vi "Sensors.vi"() -> ()   [LabVIEW 2018]
panel:
  out "Oil Pump":string
  out "Oil Pressure":string
  out "Chamber Temp":string
  out "Oil Temp":string
  out "Target Temp":string
  out "Vacuum":string
  out "-":string
  out "Recoat Temp":string
  out "Sprinkler Temp":string
  out "Overhead Temp":string
  out "Radiation Limit":string
  out "Recon Vars 2":string
  out "-":string
  out "Interlocks":string
  out "Solenoid A":string
  out "Solenoid B":string
  out "BOP 100-2ML":string
  out "Agilent 33120A":string
  out "- Grid Bias":string
  out "+ Grid Bias":string
  out "Cathode B":string
  out "Cathode C":string
  out "Cathode A":string
  out "Recon Vars":string
  out "Pulser C":string
  out "Pulser B":string
  out "Due MCU":string
  out "Pulser A":string
  out "Quantum 9530":string
  out "Beam Extraction":string
  out "Error":string
  out "Scanning Vars":string
  out "rPi Swivel Cam":string
  out "Port & Oil Cams":string
  out "Room Cams":string
  out "BeamAcceleration":string
  out "Sensors":string
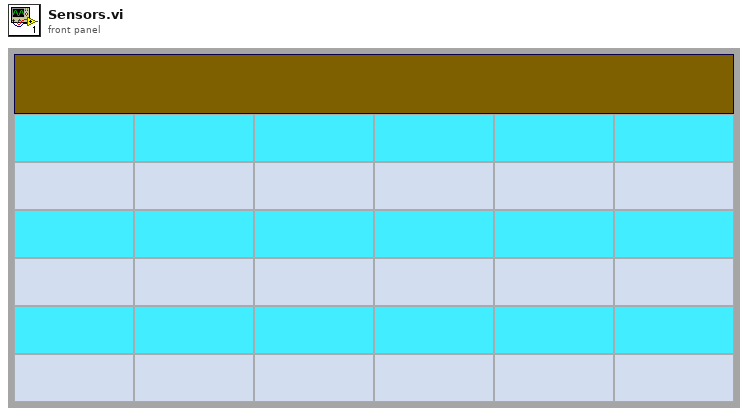
[diagram p1: front panel]
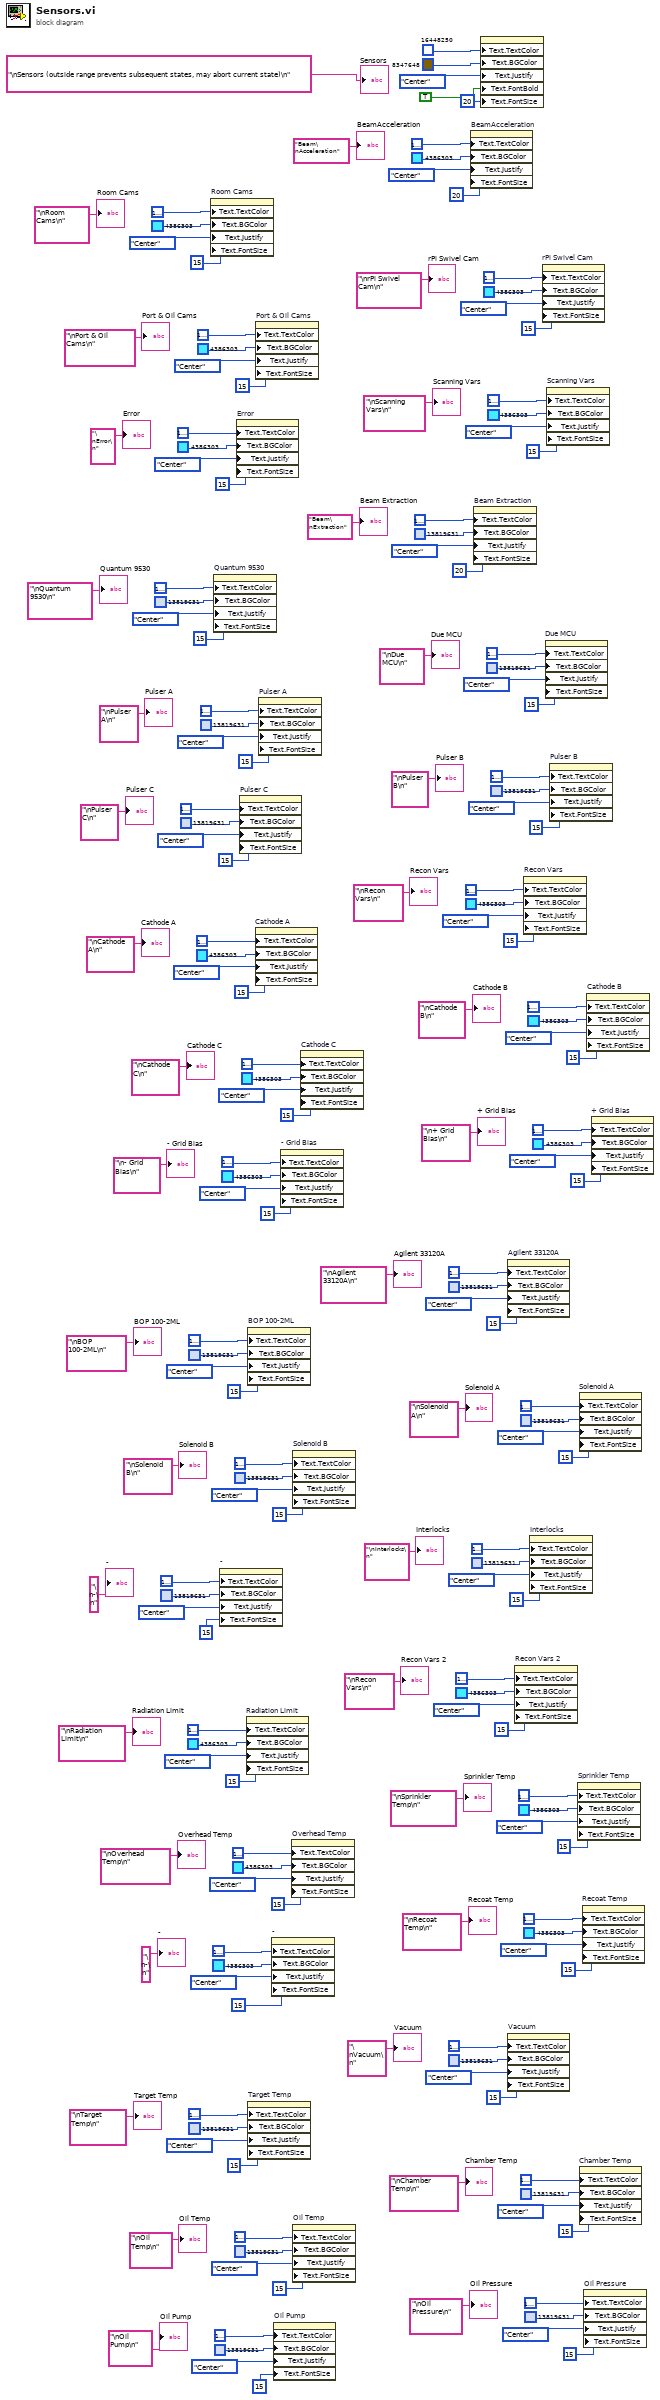
[diagram p0: block diagram]
diagram:
  n1 = property on="Room Cams" class="Str"("Text.TextColor"=u32 16777228, "Text.BGColor"=u32 4386303, "Text.Justify"=enum16{"Left", "Center", "Right"}."Center" ("Text.Justification"), "Text.FontSize"=u32 15 ("Text.Font:Size")) -> ()  [unwired: 2 in, 2 out]
  n2 = property on="Quantum 9530" class="Str"("Text.TextColor"=u32 16777228, "Text.BGColor"=u32 13819631, "Text.Justify"=enum16{"Left", "Center", "Right"}."Center" ("Text.Justification"), "Text.FontSize"=u32 15 ("Text.Font:Size")) -> ()  [unwired: 2 in, 2 out]
  n3 = property on="-" class="Str"("Text.TextColor"=u32 16777228, "Text.BGColor"=u32 13819631, "Text.Justify"=enum16{"Left", "Center", "Right"}."Center" ("Text.Justification"), "Text.FontSize"=u32 15 ("Text.Font:Size")) -> ()  [unwired: 2 in, 2 out]
  n4 = property on="Error" class="Str"("Text.TextColor"=u32 16777228, "Text.BGColor"=u32 4386303, "Text.Justify"=enum16{"Left", "Center", "Right"}."Center" ("Text.Justification"), "Text.FontSize"=u32 15 ("Text.Font:Size")) -> ()  [unwired: 2 in, 2 out]
  n5 = property on="Pulser C" class="Str"("Text.TextColor"=u32 16777228, "Text.BGColor"=u32 13819631, "Text.Justify"=enum16{"Left", "Center", "Right"}."Center" ("Text.Justification"), "Text.FontSize"=u32 15 ("Text.Font:Size")) -> ()  [unwired: 2 in, 2 out]
  n6 = property on="Radiation Limit" class="Str"("Text.TextColor"=u32 16777228, "Text.BGColor"=u32 4386303, "Text.Justify"=enum16{"Left", "Center", "Right"}."Center" ("Text.Justification"), "Text.FontSize"=u32 15 ("Text.Font:Size")) -> ()  [unwired: 2 in, 2 out]
  n7 = property on="BOP 100-2ML" class="Str"("Text.TextColor"=u32 16777228, "Text.BGColor"=u32 13819631, "Text.Justify"=enum16{"Left", "Center", "Right"}."Center" ("Text.Justification"), "Text.FontSize"=u32 15 ("Text.Font:Size")) -> ()  [unwired: 2 in, 2 out]
  n8 = property on="Target Temp" class="Str"("Text.TextColor"=u32 16777228, "Text.BGColor"=u32 13819631, "Text.Justify"=enum16{"Left", "Center", "Right"}."Center" ("Text.Justification"), "Text.FontSize"=u32 15 ("Text.Font:Size")) -> ()  [unwired: 2 in, 2 out]
  n9 = property on="Cathode A" class="Str"("Text.TextColor"=u32 16777228, "Text.BGColor"=u32 4386303, "Text.Justify"=enum16{"Left", "Center", "Right"}."Center" ("Text.Justification"), "Text.FontSize"=u32 15 ("Text.Font:Size")) -> ()  [unwired: 2 in, 2 out]
  n10 = property on="Port & Oil Cams" class="Str"("Text.TextColor"=u32 16777228, "Text.BGColor"=u32 4386303, "Text.Justify"=enum16{"Left", "Center", "Right"}."Center" ("Text.Justification"), "Text.FontSize"=u32 15 ("Text.Font:Size")) -> ()  [unwired: 2 in, 2 out]
  n11 = property on="Pulser A" class="Str"("Text.TextColor"=u32 16777228, "Text.BGColor"=u32 13819631, "Text.Justify"=enum16{"Left", "Center", "Right"}."Center" ("Text.Justification"), "Text.FontSize"=u32 15 ("Text.Font:Size")) -> ()  [unwired: 2 in, 2 out]
  n12 = property on="-" class="Str"("Text.TextColor"=u32 16777228, "Text.BGColor"=u32 4386303, "Text.Justify"=enum16{"Left", "Center", "Right"}."Center" ("Text.Justification"), "Text.FontSize"=u32 15 ("Text.Font:Size")) -> ()  [unwired: 2 in, 2 out]
  n13 = property on="Oil Pump" class="Str"("Text.TextColor"=u32 16777228, "Text.BGColor"=u32 13819631, "Text.Justify"=enum16{"Left", "Center", "Right"}."Center" ("Text.Justification"), "Text.FontSize"=u32 15 ("Text.Font:Size")) -> ()  [unwired: 2 in, 2 out]
  n14 = property on="- Grid Bias" class="Str"("Text.TextColor"=u32 16777228, "Text.BGColor"=u32 4386303, "Text.Justify"=enum16{"Left", "Center", "Right"}."Center" ("Text.Justification"), "Text.FontSize"=u32 15 ("Text.Font:Size")) -> ()  [unwired: 2 in, 2 out]
  n15 = property on="Overhead Temp" class="Str"("Text.TextColor"=u32 16777228, "Text.BGColor"=u32 4386303, "Text.Justify"=enum16{"Left", "Center", "Right"}."Center" ("Text.Justification"), "Text.FontSize"=u32 15 ("Text.Font:Size")) -> ()  [unwired: 2 in, 2 out]
  n16 = property on="Solenoid B" class="Str"("Text.TextColor"=u32 16777228, "Text.BGColor"=u32 13819631, "Text.Justify"=enum16{"Left", "Center", "Right"}."Center" ("Text.Justification"), "Text.FontSize"=u32 15 ("Text.Font:Size")) -> ()  [unwired: 2 in, 2 out]
  n17 = property on="Oil Temp" class="Str"("Text.TextColor"=u32 16777228, "Text.BGColor"=u32 13819631, "Text.Justify"=enum16{"Left", "Center", "Right"}."Center" ("Text.Justification"), "Text.FontSize"=u32 15 ("Text.Font:Size")) -> ()  [unwired: 2 in, 2 out]
  n18 = property on="Cathode C" class="Str"("Text.TextColor"=u32 16777228, "Text.BGColor"=u32 4386303, "Text.Justify"=enum16{"Left", "Center", "Right"}."Center" ("Text.Justification"), "Text.FontSize"=u32 15 ("Text.Font:Size")) -> ()  [unwired: 2 in, 2 out]
  n19 = property on="BeamAcceleration" class="Str"("Text.TextColor"=u32 16777228, "Text.BGColor"=u32 4386303, "Text.Justify"=enum16{"Left", "Center", "Right"}."Center" ("Text.Justification"), "Text.FontSize"=u32 20 ("Text.Font:Size")) -> ()  [unwired: 2 in, 2 out]
  n20 = property on="Beam Extraction" class="Str"("Text.TextColor"=u32 16777228, "Text.BGColor"=u32 13819631, "Text.Justify"=enum16{"Left", "Center", "Right"}."Center" ("Text.Justification"), "Text.FontSize"=u32 20 ("Text.Font:Size")) -> ()  [unwired: 2 in, 2 out]
  n21 = property on="Sensors" class="Str"("Text.TextColor"=u32 16448250, "Text.BGColor"=u32 8347648, "Text.Justify"=enum16{"Left", "Center", "Right"}."Center" ("Text.Justification"), "Text.FontBold"=TRUE ("Text.Font:Bold"), "Text.FontSize"=u32 20 ("Text.Font:Size")) -> ()  [unwired: 2 in, 2 out]
  n22 = property on="Agilent 33120A" class="Str"("Text.TextColor"=u32 16777228, "Text.BGColor"=u32 13819631, "Text.Justify"=enum16{"Left", "Center", "Right"}."Center" ("Text.Justification"), "Text.FontSize"=u32 15 ("Text.Font:Size")) -> ()  [unwired: 2 in, 2 out]
  n23 = property on="Vacuum" class="Str"("Text.TextColor"=u32 16777228, "Text.BGColor"=u32 13819631, "Text.Justify"=enum16{"Left", "Center", "Right"}."Center" ("Text.Justification"), "Text.FontSize"=u32 15 ("Text.Font:Size")) -> ()  [unwired: 2 in, 2 out]
  n24 = property on="Recon Vars 2" class="Str"("Text.TextColor"=u32 16777228, "Text.BGColor"=u32 4386303, "Text.Justify"=enum16{"Left", "Center", "Right"}."Center" ("Text.Justification"), "Text.FontSize"=u32 15 ("Text.Font:Size")) -> ()  [unwired: 2 in, 2 out]
  n25 = property on="Recon Vars" class="Str"("Text.TextColor"=u32 16777228, "Text.BGColor"=u32 4386303, "Text.Justify"=enum16{"Left", "Center", "Right"}."Center" ("Text.Justification"), "Text.FontSize"=u32 15 ("Text.Font:Size")) -> ()  [unwired: 2 in, 2 out]
  n26 = property on="Interlocks" class="Str"("Text.TextColor"=u32 16777228, "Text.BGColor"=u32 13819631, "Text.Justify"=enum16{"Left", "Center", "Right"}."Center" ("Text.Justification"), "Text.FontSize"=u32 15 ("Text.Font:Size")) -> ()  [unwired: 2 in, 2 out]
  n27 = property on="rPi Swivel Cam" class="Str"("Text.TextColor"=u32 16777228, "Text.BGColor"=u32 4386303, "Text.Justify"=enum16{"Left", "Center", "Right"}."Center" ("Text.Justification"), "Text.FontSize"=u32 15 ("Text.Font:Size")) -> ()  [unwired: 2 in, 2 out]
  n28 = property on="Due MCU" class="Str"("Text.TextColor"=u32 16777228, "Text.BGColor"=u32 13819631, "Text.Justify"=enum16{"Left", "Center", "Right"}."Center" ("Text.Justification"), "Text.FontSize"=u32 15 ("Text.Font:Size")) -> ()  [unwired: 2 in, 2 out]
  n29 = property on="Scanning Vars" class="Str"("Text.TextColor"=u32 16777228, "Text.BGColor"=u32 4386303, "Text.Justify"=enum16{"Left", "Center", "Right"}."Center" ("Text.Justification"), "Text.FontSize"=u32 15 ("Text.Font:Size")) -> ()  [unwired: 2 in, 2 out]
  n30 = property on="Pulser B" class="Str"("Text.TextColor"=u32 16777228, "Text.BGColor"=u32 13819631, "Text.Justify"=enum16{"Left", "Center", "Right"}."Center" ("Text.Justification"), "Text.FontSize"=u32 15 ("Text.Font:Size")) -> ()  [unwired: 2 in, 2 out]
  n31 = property on="Sprinkler Temp" class="Str"("Text.TextColor"=u32 16777228, "Text.BGColor"=u32 4386303, "Text.Justify"=enum16{"Left", "Center", "Right"}."Center" ("Text.Justification"), "Text.FontSize"=u32 15 ("Text.Font:Size")) -> ()  [unwired: 2 in, 2 out]
  n32 = property on="Solenoid A" class="Str"("Text.TextColor"=u32 16777228, "Text.BGColor"=u32 13819631, "Text.Justify"=enum16{"Left", "Center", "Right"}."Center" ("Text.Justification"), "Text.FontSize"=u32 15 ("Text.Font:Size")) -> ()  [unwired: 2 in, 2 out]
  n33 = property on="Chamber Temp" class="Str"("Text.TextColor"=u32 16777228, "Text.BGColor"=u32 13819631, "Text.Justify"=enum16{"Left", "Center", "Right"}."Center" ("Text.Justification"), "Text.FontSize"=u32 15 ("Text.Font:Size")) -> ()  [unwired: 2 in, 2 out]
  n34 = property on="Recoat Temp" class="Str"("Text.TextColor"=u32 16777228, "Text.BGColor"=u32 4386303, "Text.Justify"=enum16{"Left", "Center", "Right"}."Center" ("Text.Justification"), "Text.FontSize"=u32 15 ("Text.Font:Size")) -> ()  [unwired: 2 in, 2 out]
  n35 = property on="Oil Pressure" class="Str"("Text.TextColor"=u32 16777228, "Text.BGColor"=u32 13819631, "Text.Justify"=enum16{"Left", "Center", "Right"}."Center" ("Text.Justification"), "Text.FontSize"=u32 15 ("Text.Font:Size")) -> ()  [unwired: 2 in, 2 out]
  n36 = property on="Cathode B" class="Str"("Text.TextColor"=u32 16777228, "Text.BGColor"=u32 4386303, "Text.Justify"=enum16{"Left", "Center", "Right"}."Center" ("Text.Justification"), "Text.FontSize"=u32 15 ("Text.Font:Size")) -> ()  [unwired: 2 in, 2 out]
  n37 = property on="+ Grid Bias" class="Str"("Text.TextColor"=u32 16777228, "Text.BGColor"=u32 4386303, "Text.Justify"=enum16{"Left", "Center", "Right"}."Center" ("Text.Justification"), "Text.FontSize"=u32 15 ("Text.Font:Size")) -> ()  [unwired: 2 in, 2 out]
  "Sensors" <- "\nSensors (outside range prevents subsequent states, may abort current state)\n" ("String")
  "BeamAcceleration" <- "Beam\nAcceleration" ("String 2")
  "Room Cams" <- "\nRoom Cams\n" ("String 2")
  "Port & Oil Cams" <- "\nPort & Oil Cams\n" ("String 2")
  "rPi Swivel Cam" <- "\nrPi Swivel Cam\n" ("String 2")
  "Scanning Vars" <- "\nScanning Vars\n" ("String 2")
  "Error" <- "\nError\n" ("String 2")
  "Beam Extraction" <- "Beam\nExtraction" ("String 2")
  "Quantum 9530" <- "\nQuantum 9530\n" ("String 2")
  "Pulser A" <- "\nPulser A\n" ("String 2")
  "Due MCU" <- "\nDue MCU\n" ("String 2")
  "Pulser B" <- "\nPulser B\n" ("String 2")
  "Pulser C" <- "\nPulser C\n" ("String 2")
  "Recon Vars" <- "\nRecon Vars\n" ("String 2")
  "Cathode A" <- "\nCathode A\n" ("String 2")
  "Cathode C" <- "\nCathode C\n" ("String 2")
  "Cathode B" <- "\nCathode B\n" ("String 2")
  "+ Grid Bias" <- "\n+ Grid Bias\n" ("String 2")
  "- Grid Bias" <- "\n- Grid Bias\n" ("String 2")
  "Agilent 33120A" <- "\nAgilent 33120A\n" ("String 2")
  "BOP 100-2ML" <- "\nBOP 100-2ML\n" ("String 2")
  "Solenoid B" <- "\nSolenoid B\n" ("String 2")
  "Solenoid A" <- "\nSolenoid A\n" ("String 2")
  "Interlocks" <- "\nInterlocks\n" ("String 2")
  "-" <- "\n-\n" ("String 2")
  "Recon Vars 2" <- "\nRecon Vars\n" ("String 2")
  "Radiation Limit" <- "\nRadiation Limit\n" ("String 2")
  "Overhead Temp" <- "\nOverhead Temp\n" ("String 2")
  "Sprinkler Temp" <- "\nSprinkler Temp\n" ("String 2")
  "Recoat Temp" <- "\nRecoat Temp\n" ("String 2")
  "-" <- "\n-\n" ("String 2")
  "Vacuum" <- "\nVacuum\n" ("String 2")
  "Target Temp" <- "\nTarget Temp\n" ("String 2")
  "Oil Temp" <- "\nOil Temp\n" ("String 2")
  "Chamber Temp" <- "\nChamber Temp\n" ("String 2")
  "Oil Pressure" <- "\nOil Pressure\n" ("String 2")
  "Oil Pump" <- "\nOil Pump\n" ("String 2")
